vi "SimpleGit Setting Dialog.vi"(8 "error in":errorcluster) -> (0 "error out":errorcluster)   [LabVIEW 2017]
uses:
  <resource>/dialog/lvconfig.llb/LV Config Write Pathlist.vi
  <resource>/dialog/lvconfig.llb/LV Config Write String.vi
panel:
  in  "DailyBranch Prefix":string
  in  "TortoiseGitProc Path":path
  in  "OK":bool
  in  "Cancel":bool
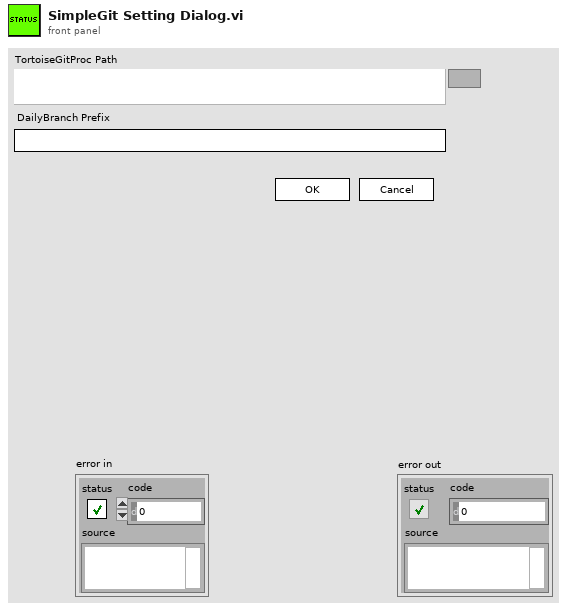
[diagram p1: front panel]
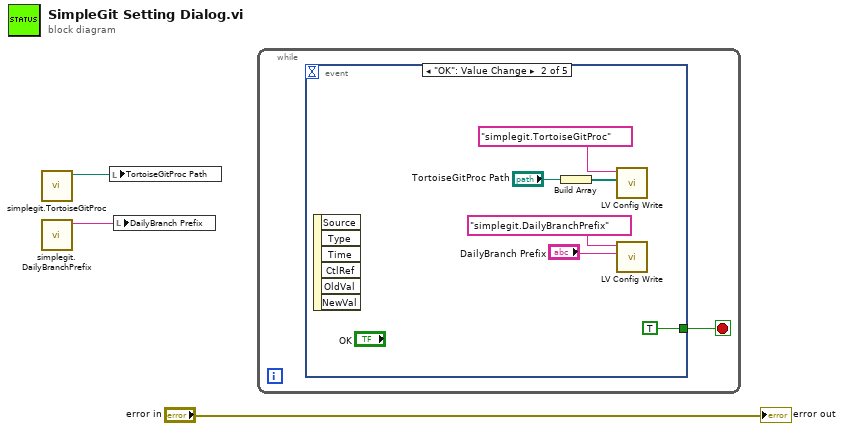
[diagram p0: block diagram]
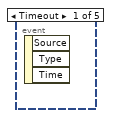
[diagram p2: hidden frame]
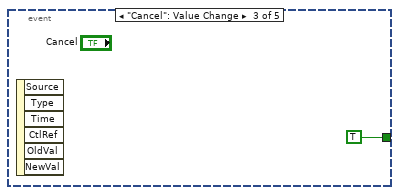
[diagram p3: hidden frame]
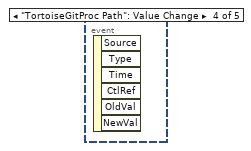
[diagram p4: hidden frame]
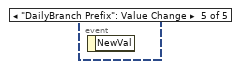
[diagram p5: hidden frame]
diagram:
  n1 = call "simplegit.TortoiseGitProc.vi"() -> ("Path"=w2:path)  [unwired: 11 in]
  n2 = call "simplegit.DailyBranchPrefix.vi"() -> ("value"=w1:string)  [unwired: 11 in]
  n3 = local write "TortoiseGitProc Path"(w2) -> ()
  n4 = local write "DailyBranch Prefix"(w1) -> ()
  n5 = while {
    stop <- w4 stop-if-true
    n6 = event shown="[1] \"OK\": Value Change" {
      selector: _ -> [_ _ _ _ _]
      dyn-events: _ -> [_ _ _ _ _]
      timeout: _ -> [_ _ _ _ _]
      tunnel: [_ TRUE TRUE _ _] -> w4
      event Timeout {
        n7 = event-data() -> ()  [unwired: 1 in, 3 out]
      }
      event "OK": Value Change {
        n8 = event-data() -> ()  [unwired: 1 in, 6 out]
        n9 = Build Array("TortoiseGitProc Path") -> (w6:path[])
        n10 = call-poly <resource>:"LV Config Write.vi"("value"=w6, "key"="simplegit.TortoiseGitProc") -> ()  [unwired: 5 in, 1 out]
        n11 = call-poly <resource>:"LV Config Write.vi"("value"="DailyBranch Prefix", "key"="simplegit.DailyBranchPrefix") -> ()  [unwired: 5 in, 1 out]
      }
      event "Cancel": Value Change {
        n12 = event-data() -> ()  [unwired: 1 in, 6 out]
      }
      event "TortoiseGitProc Path": Value Change {
        n13 = event-data() -> ()  [unwired: 1 in, 6 out]
      }
      event "DailyBranch Prefix": Value Change {
        n14 = event-data() -> ()  [unwired: 1 in, 1 out]
      }
    }
  }
  "error out" <- "error in"
